vi "Wait_for_blank_buffer.vi"(8 "error in (no error)":errorcluster, 11 "VISA Refnum in":refnum<visa-resource-name>) -> (0 "error out":errorcluster, 3 "VISA Refnum out":refnum<visa-resource-name>)   [LabVIEW 2017]
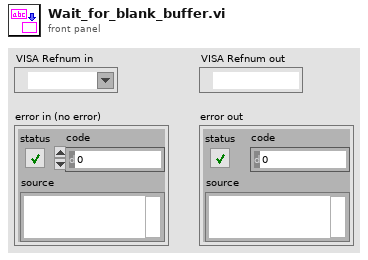
[diagram p1: front panel]
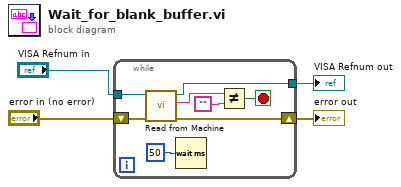
[diagram p0: block diagram]
diagram:
  n1 = while {
    tunnel: "VISA Refnum in" -> [w12]
    shift-right: [w7] -> w4
    shift-left: "error in (no error)" -> [w11]
    tunnel: [w6] -> w3
    stop <- w9 stop-if-true
    n2 = call "Read from Machine.vi"("error in (no error)"=w11, "Machine In"=w12) -> ("error out"=w7:errorcluster, "read buffer"=w8:string, "Machine Out"=w6:refnum<visa-resource-name>)  [unwired: 7 in]
    n3 = Wait (ms)(milliseconds to wait=u32 50) -> ()  [unwired: 1 out]
    n4 = Not Equal?(x=w8, y="") -> (x != y?=w9:bool)
  }
  "error out" <- w4
  "VISA Refnum out" <- w3
